vi "Convert FPS to Counts per 100ms.vi"(5 "RevMotor/RevWheel":dbl=6.67 format="%#_13g", 7 "Wheel Diameter (in)":dbl=4.0 format="%#_13g", 10 "Velocity PPR":dbl=6.67 format="%#_13g", 11 "Translation Speed (ft/s)":dbl) -> (3 "Motor Speed (Counts/100ms) Out":dbl)   [LabVIEW 2023, in "Thor-SwerveDrive_ACT.lvlib"]
uses:
  Thor-SwerveDrive_ACT.lvlib
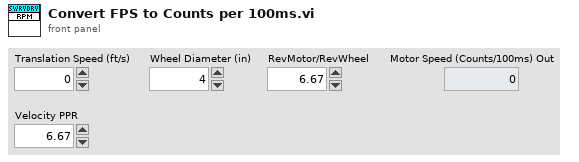
[diagram p1: front panel]
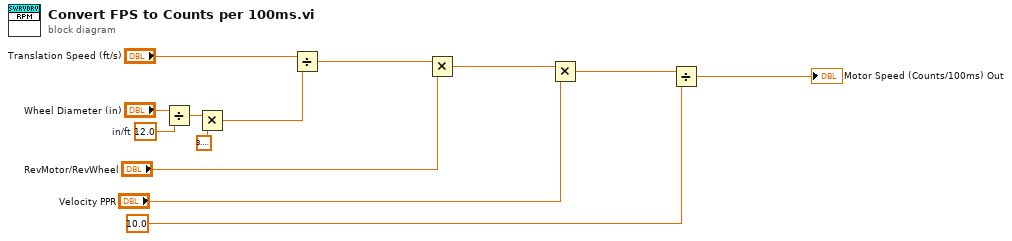
[diagram p0: block diagram]
diagram:
  w12 = 12.0  # in/ft
  n1 = Divide(x="Wheel Diameter (in)", y=w12) -> (x/y=w10:dbl)
  n2 = Multiply(x=w10, y=3.141592653589793) -> (x*y=w9:dbl)
  n3 = Divide(x="Translation Speed (ft/s)", y=w9) -> (x/y=w5:dbl)
  n4 = Multiply(x=w5, y="RevMotor/RevWheel") -> (x*y=w6:dbl)
  n5 = Multiply(x=w6, y="Velocity PPR") -> (x*y=w4:dbl)
  n6 = Divide(x=w4, y=10.0) -> (x/y=→"Motor Speed (Counts/100ms) Out":dbl)
